vi "Helper SubVI - Mode Check.vi"(6 "sample freq":dbl=1.0, 8 "freq range":cluster{"high":dbl, "low":dbl}, 11 "frequency components":T1(array[cluster])) -> (0 "phase":dbl[][](array[numeric]), 1 "mag":dbl[][](array[numeric]), 2 "damping factor":dbl[](array[numeric]), 3 "freq":dbl[](array[numeric]))   [LabVIEW 2023]
doc: "Returns the frequency components whose frequencies are in a specified frequency range."
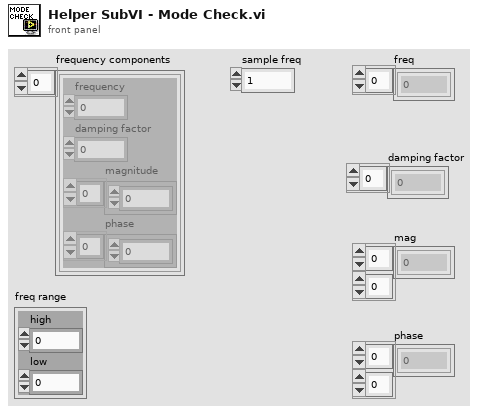
[diagram p1: front panel]
types:
  T1 = cluster{"frequency":dbl, "damping factor":dbl, "magnitude":dbl[], "phase":dbl[]}[]
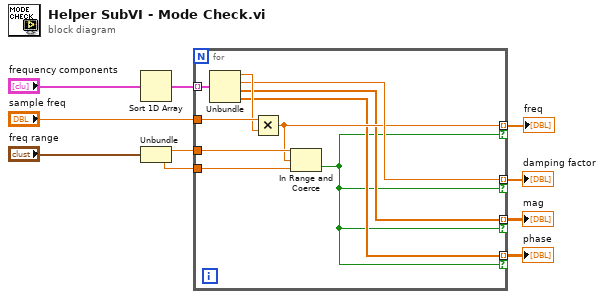
[diagram p0: block diagram]
diagram:
  n1 = Sort 1D Array(array="frequency components") -> (sorted array=w7:T1)
  n2 = Unbundle("freq range") -> ("high"=w9:dbl, "low"=w8:dbl)
  n3 = for {
    tunnel: w7 -> [w20] mode=indexing
    tunnel: w9 -> [w19]
    tunnel: w8 -> [w18]
    tunnel: "sample freq" -> [w17]
    tunnel: [w15] -> w3 mode=indexing if=w11
    tunnel: [w14] -> w4 mode=indexing if=w11
    tunnel: [w13] -> w2 mode=indexing if=w11
    tunnel: [w12] -> w1 mode=indexing if=w11
    n4 = Unbundle(w20) -> ("frequency"=w16:dbl, "damping factor"=w15:dbl, "magnitude"=w13:dbl[], "phase"=w12:dbl[])
    n5 = Multiply(x=w17, y=w16) -> (x*y=w14:dbl)
    n6 = In Range and Coerce(upper limit=w19, x=w14, lower limit=w18) -> (In Range?=w11:bool)  [unwired: 1 out]
  }
  "phase" <- w1
  "mag" <- w2
  "damping factor" <- w3
  "freq" <- w4
